vi "aw_GetData.vi"(6 "x-nem-datetime":string, 8 "error in":errorcluster, 9 "pwd":string, 10 "User":string, 11 "URL":string) -> (0 "error out":errorcluster, 2 "Response JSON":string, 3 "Response headers":string)   [LabVIEW 2015, in "AuraWheel.lvlib"]
uses:
  AuraWheel.lvlib
  <vilib>/httpClient/LabVIEWHTTPClient.lvlib
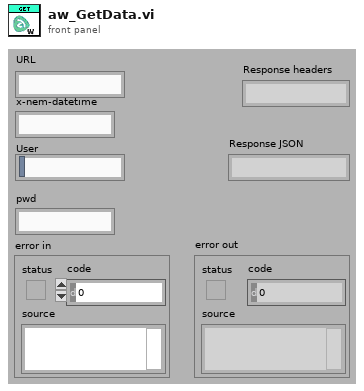
[diagram p1: front panel]
types:
  T1 = typedef "LabVIEWHTTPClient.lvlib/ClientHandle.ctl" = refnum<k1>
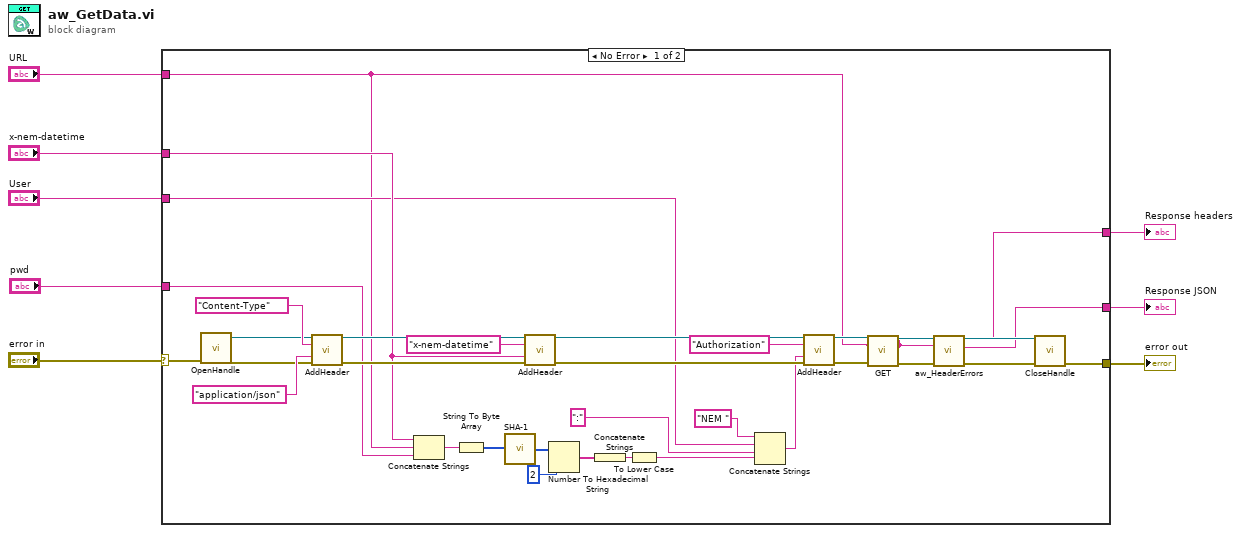
[diagram p0: block diagram]
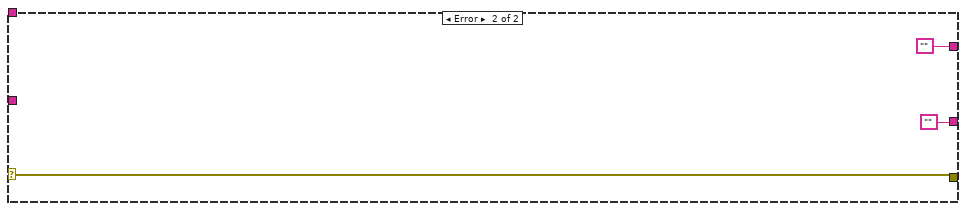
[diagram p2: hidden frame]
diagram:
  n1 = case shown="No Error" "error in" {
    selector: "error in" -> [w27 w45]
    tunnel: "x-nem-datetime" -> [w28 _]
    tunnel: [w26 w45] -> w6
    tunnel: "URL" -> [w16 _]
    tunnel: "User" -> [w22 _]
    tunnel: "pwd" -> [w17 _]
    tunnel: [w12 ""] -> w2
    tunnel: [w13 ""] -> w1
    frame No Error {
      n2 = call <vilib>:"OpenHandle.vi"("error in (no error)"=w27) -> ("client handle out"=w30:T1, "error out"=w31:errorcluster)  [unwired: 13 in]
      n3 = call <vilib>:"AddHeader.vi"("client handle"=w30, "header"="Content-Type", "value"="application/json", "error in (no error)"=w31) -> ("client handle out"=w42:T1, "error out"=w41:errorcluster)  [unwired: 10 in]
      n4 = Concatenate Strings(w28, w16, w17) -> (w36:string)
      n5 = String To Byte Array(string=w36) -> (unsigned byte array=w35:u8[])
      n6 = call "SHA-1.vi"("Data"=w35) -> ("message-digest"=w34:u8[])
      n7 = call <vilib>:"AddHeader.vi"("client handle"=w42, "header"="x-nem-datetime" ("value"), "value"=w28, "error in (no error)"=w41) -> ("client handle out"=w39:T1, "error out"=w38:errorcluster)  [unwired: 10 in]
      n8 = Number To Hexadecimal String(1:i16 2 ("width (-)"), 2:w34) -> (0:w33:string[])
      n9 = Concatenate Strings(w33) -> (w19:string)
      n10 = To Lower Case(string=w19) -> (all lower case string=w18:string)
      n11 = Concatenate Strings("NEM " ("string"), w22, ":" ("string"), w18) -> (w11:string)
      n12 = call <vilib>:"AddHeader.vi"("client handle"=w39, "header"="Authorization" ("value"), "value"=w11, "error in (no error)"=w38) -> ("client handle out"=w24:T1, "error out"=w25:errorcluster)  [unwired: 10 in]
      n13 = call <vilib>:"GET.vi"("client handle"=w24, "url"=w16, "error in (no error)"=w25) -> ("client handle out"=w23:T1, "headers"=w9:string, "error out"=w15:errorcluster)  [unwired: 9 in, 1 out]
      n14 = call "aw_HeaderErrors.vi"("error in"=w15, "Response Body"=w9, "Response Headers"=w9) -> ("error out"=w14:errorcluster, "Response Body Out"=w13:string, "Response Headers Out"=w12:string)  [unwired: 6 in]
      n15 = call <vilib>:"CloseHandle.vi"("client handle"=w23, "error in (no error)"=w14) -> ("error out"=w26:errorcluster)  [unwired: 13 in]
    }
    frame Error {
    }
  }
  "error out" <- w6
  "Response headers" <- w2
  "Response JSON" <- w1
